vi "manual test UI.vi"(8 "error in (no error)":errorcluster caption="Fehler (Eingang, kein Fehler)", 11 "Spannungseinbruch Eingang":refnum<class "Spannungseinbruch.lvclass"> caption="DNL_LabVIEW Object in") -> (0 "error out":errorcluster caption="Fehler (Ausgang)", 1 "abbrechen":bool, 2 "Parameters":u32[](array[numeric]), 3 "Spannungseinbruch Ausgang":refnum<class "Spannungseinbruch.lvclass"> caption="DNL_LabVIEW Object out")   [LabVIEW 2013, in "Spannungseinbruch.lvclass"]
uses:
  Spannungseinbruch.lvclass
  Devices/CEG4500/ceg_make_cutofftest_states.ctl
panel:
  out "parameters":string[](array[string])
  in  "Parameters 2":u32[](array[numeric])
  in  "Testbeschreibung":string
  out "col":i32=3
  in  "abbrechen":bool
  in  "0 2":bool=TRUE
  in  "315 2":bool=TRUE
  in  "270 2":bool=TRUE
  in  "225 2":bool=TRUE
  in  "180 2":bool=TRUE
  in  "135 2":bool=TRUE
  in  "90 2":bool=TRUE
  in  "45 2":bool=TRUE
  in  "500ms 2":bool=TRUE
  in  "200ms 2":bool=TRUE
  in  "20ms 2":bool=TRUE
  in  "5000ms 2":bool=TRUE
  in  "erstellen":bool
  in  "COUNTER (1 - 999)":i32=5 min=0 max=999
  out "Str_counter":string
  in  "REP TIME (1-999s)":i32 min=1 max=999
  out "Str_reptime":string
  out "Commandlist":string
  out "parameter table":string[][](table)
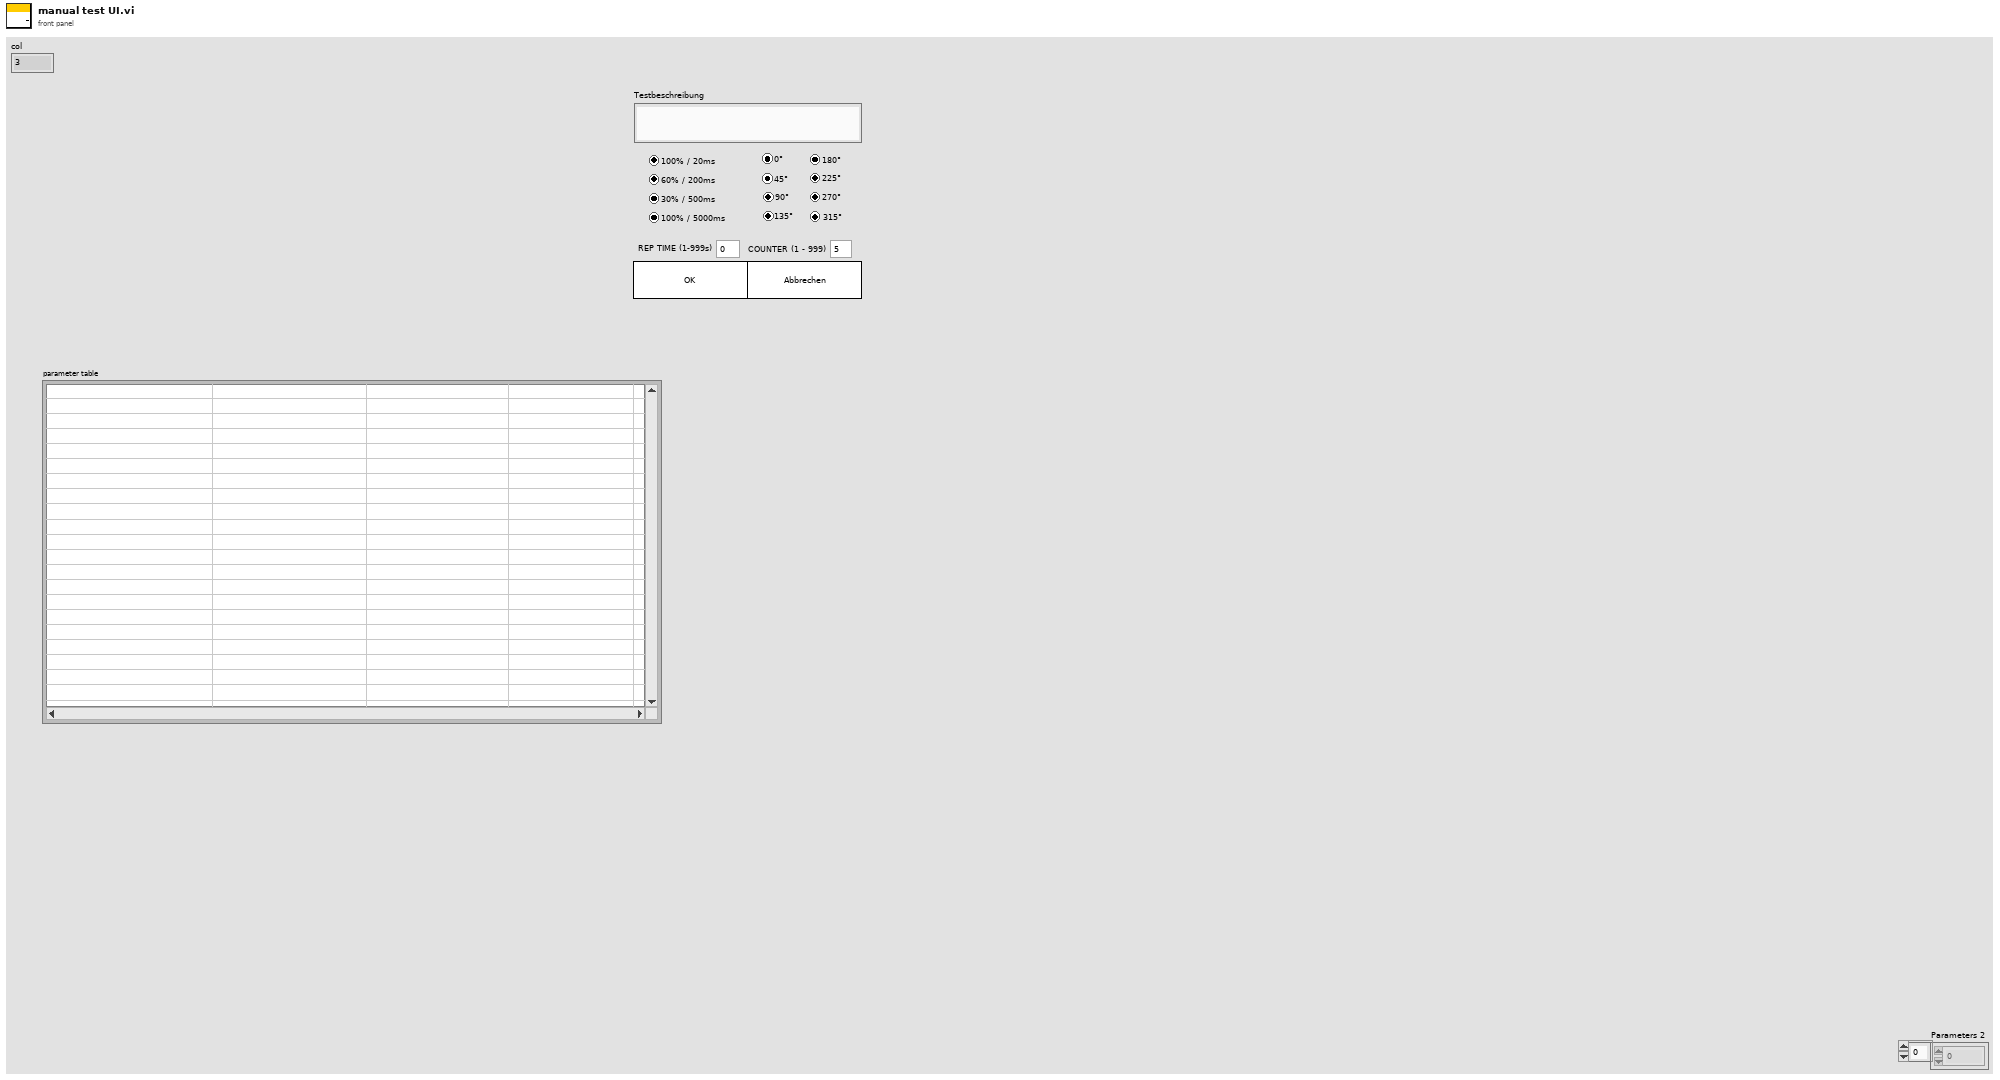
[diagram p1: front panel]
types:
  T1 = typedef "Spannungseinbruch.lvclass/ceg_make_cutofftest_states.ctl" = enum16{"make last test", "end", "make cmd strings", "make num strings", "start"}
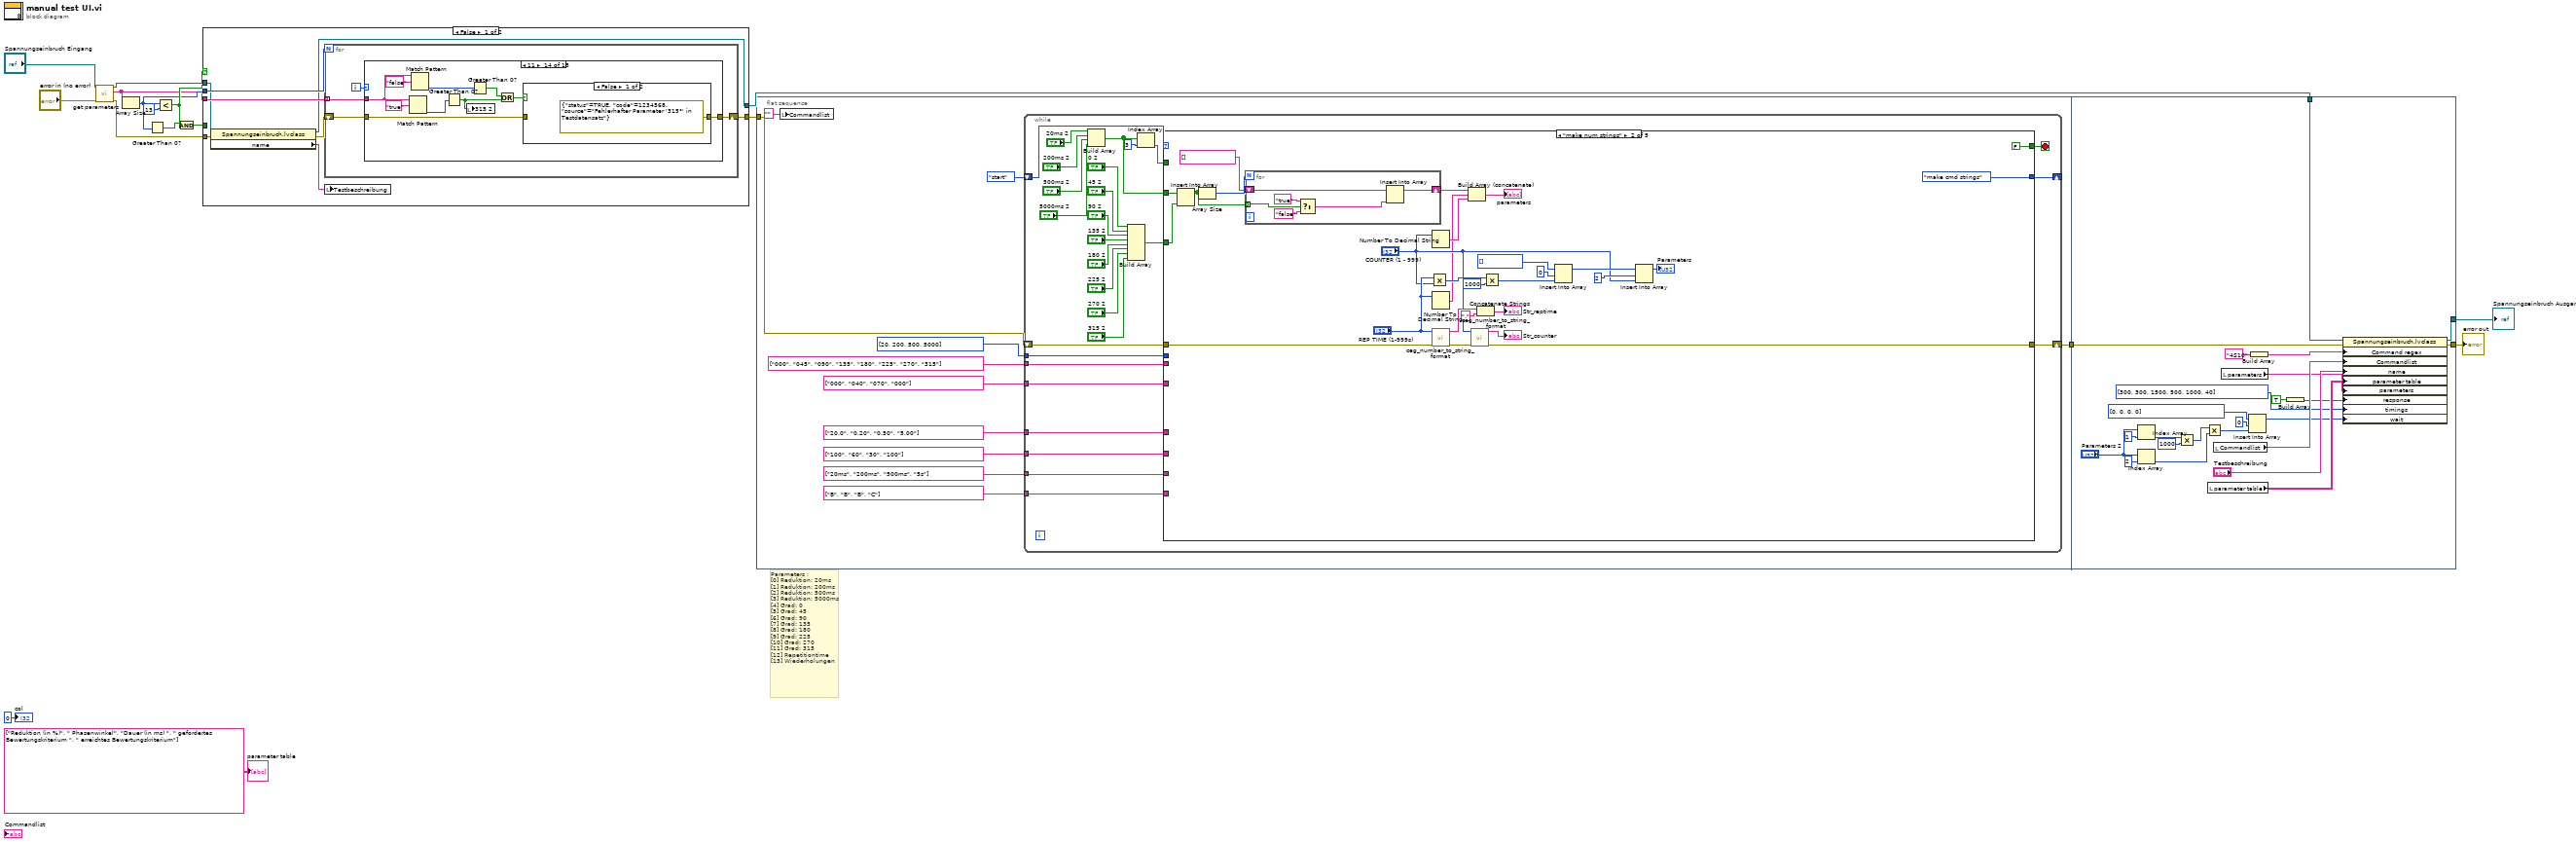
[diagram p0: block diagram]
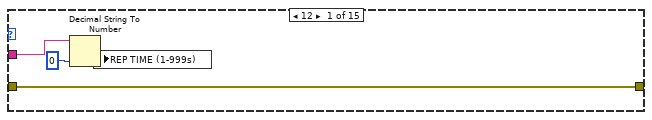
[diagram p2: hidden frame]
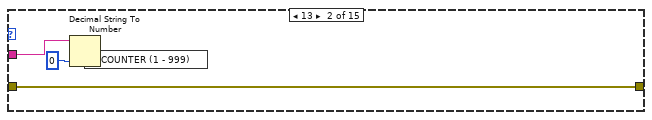
[diagram p3: hidden frame]
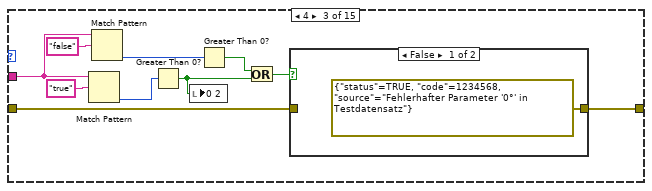
[diagram p4: hidden frame]
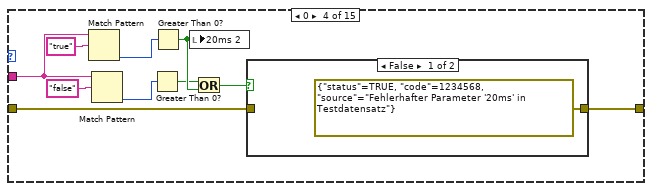
[diagram p6: hidden frame]
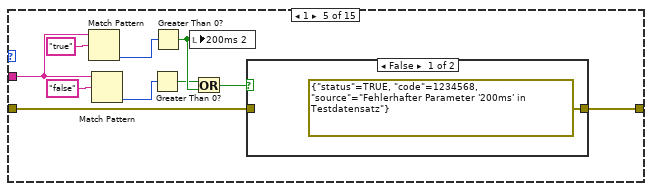
[diagram p8: hidden frame]
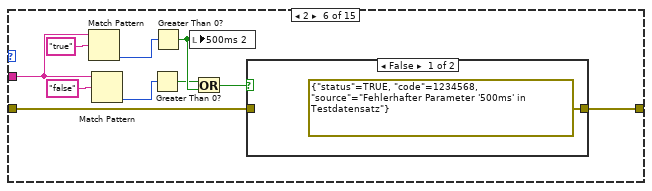
[diagram p10: hidden frame]
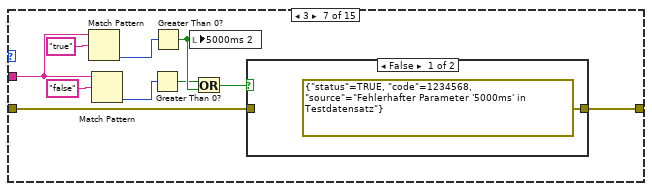
[diagram p12: hidden frame]
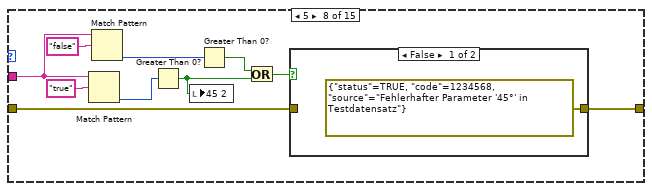
[diagram p14: hidden frame]
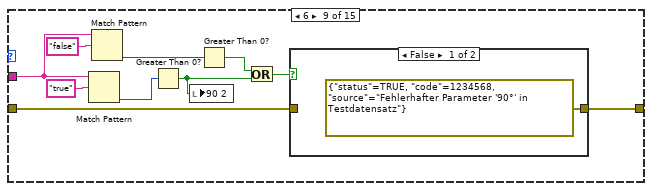
[diagram p16: hidden frame]
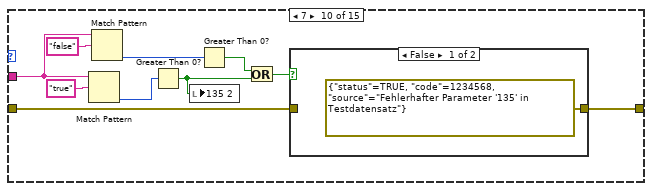
[diagram p18: hidden frame]
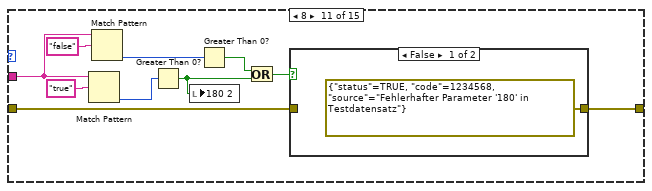
[diagram p20: hidden frame]
diagram:
  # "Parameters :\n[0] Reduktion: 20ms\n[1] Reduktion: 200ms\n[2] Reduktion: 500ms\n[3] Reduktion: 5000ms\n[4] Grad: 0\n[5] Grad: 45\n[6] Grad: 90\n[7] Grad: 135\n[8] Grad: 180\n[9] Grad: 225\n[10] Grad: 270\n[11] Grad: 315\n[12] Repetitiontime\n[13] Wiederholungen"
  n1 = call-dynamic "get parameters.vi"("error in (no error)"="error in (no error)", "TestInterface (Eingang)"="Spannungseinbruch Eingang") -> ("error out"=w7:errorcluster, "parameters"=w6:string[], "TestInterface (Ausgang)"=w13:refnum<class "Spannungseinbruch.lvclass">)  [unwired: 7 in]
  n2 = Array Size(array=w6) -> (size(s)=w9:i32)
  n3 = Greater Than 0?(x=w9) -> (x > 0?=w10:bool)
  n4 = Less?(x=w9, y=13) -> (x < y?=w11:bool)
  n5 = And(x=w10, y=w11) -> (x .and. y?=w12:bool)
  n6 = case shown="False" w11 {
    tunnel: w9 -> [w25 _]
    tunnel: w6 -> [w24 _]
    tunnel: w7 -> [w21 w186]
    tunnel: [w23 w184] -> w1
    tunnel: w12 -> [_ w185]
    tunnel: w13 -> [w22 w183]
    tunnel: [w18 w183] -> w3
    frame False {
      n7 = property class="Spannungseinbruch.lvclass"(reference=w22, error in=w21) -> (reference out=w18:refnum<class "Spannungseinbruch.lvclass">, error out=w20:errorcluster, "name"=w19:string)
      n8 = for {
        N: w25 -> [_]
        tunnel: w24 -> [w28] mode=indexing
        shift-right: [w27] -> w23
        shift-left: w20 -> [w26]
        i -> [w29]
        n9 = case shown="11" w29 {
          tunnel: w28 -> [w33 w37 w38 w50 w62 w74 w86 w98 w110 w122 w134 w146 w158 w170 _]
          tunnel: w26 -> [w30 w34 w40 w52 w64 w76 w88 w100 w112 w124 w136 w148 w160 w172 _]
          tunnel: [w30 w34 w42 w54 w66 w78 w90 w102 w114 w126 w138 w150 w162 w174 errorcluster {"status"=TRUE, "code"=1234567, "source"="zu viele Parameter für Test"} ("error constant")] -> w27
          frame 12 {
            n10 = Decimal String To Number(string=w33, default (0L)=u32 0 ("default (0 I32)")) -> (number=w32:u32)  [unwired: 1 in, 1 out]
            n11 = local write "REP TIME (1-999s)"(w32) -> ()
          }
          frame 13 {
            n12 = Decimal String To Number(string=w37, default (0L)=u32 0 ("default (0 I32)")) -> (number=w36:u32)  [unwired: 1 in, 1 out]
            n13 = local write "COUNTER (1 - 999)"(w36) -> ()
          }
          frame 4 {
            n14 = Match Pattern(string=w38, regular expression="true") -> (offset past match=w46:i32)  [unwired: 1 in, 3 out]
            n15 = Match Pattern(string=w38, regular expression="false") -> (offset past match=w44:i32)  [unwired: 1 in, 3 out]
            n16 = Greater Than 0?(x=w46) -> (x > 0?=w43:bool)
            n17 = local write "0 2"(w43) -> ()
            n18 = Greater Than 0?(x=w44) -> (x > 0?=w41:bool)
            n19 = Or(x=w41, y=w43) -> (x .or. y?=w39:bool)
            n20 = case shown="False" w39 {
              tunnel: [errorcluster {"status"=TRUE, "code"=1234568, "source"="Fehlerhafter Parameter '0°' in Testdatensatz"} ("error constant") w49] -> w42
              tunnel: w40 -> [_ w49]
              frame False {
              }
              frame True {
              }
            }
          }
          frame 0 {
            n21 = Match Pattern(string=w50, regular expression="true") -> (offset past match=w58:i32)  [unwired: 1 in, 3 out]
            n22 = Match Pattern(string=w50, regular expression="false") -> (offset past match=w56:i32)  [unwired: 1 in, 3 out]
            n23 = Greater Than 0?(x=w56) -> (x > 0?=w53:bool)
            n24 = Greater Than 0?(x=w58) -> (x > 0?=w55:bool)
            n25 = local write "20ms 2"(w55) -> ()
            n26 = Or(x=w53, y=w55) -> (x .or. y?=w51:bool)
            n27 = case shown="False" w51 {
              tunnel: [errorcluster {"status"=TRUE, "code"=1234568, "source"="Fehlerhafter Parameter '20ms' in Testdatensatz"} ("error constant") w61] -> w54
              tunnel: w52 -> [_ w61]
              frame False {
              }
              frame True {
              }
            }
          }
          frame 1 {
            n28 = Match Pattern(string=w62, regular expression="true") -> (offset past match=w70:i32)  [unwired: 1 in, 3 out]
            n29 = Match Pattern(string=w62, regular expression="false") -> (offset past match=w68:i32)  [unwired: 1 in, 3 out]
            n30 = Greater Than 0?(x=w68) -> (x > 0?=w65:bool)
            n31 = Greater Than 0?(x=w70) -> (x > 0?=w67:bool)
            n32 = local write "200ms 2"(w67) -> ()
            n33 = Or(x=w65, y=w67) -> (x .or. y?=w63:bool)
            n34 = case shown="False" w63 {
              tunnel: [errorcluster {"status"=TRUE, "code"=1234568, "source"="Fehlerhafter Parameter '200ms' in Testdatensatz"} ("error constant") w73] -> w66
              tunnel: w64 -> [_ w73]
              frame False {
              }
              frame True {
              }
            }
          }
          frame 2 {
            n35 = Match Pattern(string=w74, regular expression="true") -> (offset past match=w82:i32)  [unwired: 1 in, 3 out]
            n36 = Match Pattern(string=w74, regular expression="false") -> (offset past match=w80:i32)  [unwired: 1 in, 3 out]
            n37 = Greater Than 0?(x=w80) -> (x > 0?=w77:bool)
            n38 = Greater Than 0?(x=w82) -> (x > 0?=w79:bool)
            n39 = local write "500ms 2"(w79) -> ()
            n40 = Or(x=w77, y=w79) -> (x .or. y?=w75:bool)
            n41 = case shown="False" w75 {
              tunnel: [errorcluster {"status"=TRUE, "code"=1234568, "source"="Fehlerhafter Parameter '500ms' in Testdatensatz"} ("error constant") w85] -> w78
              tunnel: w76 -> [_ w85]
              frame False {
              }
              frame True {
              }
            }
          }
          frame 3 {
            n42 = Match Pattern(string=w86, regular expression="true") -> (offset past match=w94:i32)  [unwired: 1 in, 3 out]
            n43 = Match Pattern(string=w86, regular expression="false") -> (offset past match=w92:i32)  [unwired: 1 in, 3 out]
            n44 = Greater Than 0?(x=w92) -> (x > 0?=w89:bool)
            n45 = Greater Than 0?(x=w94) -> (x > 0?=w91:bool)
            n46 = local write "5000ms 2"(w91) -> ()
            n47 = Or(x=w89, y=w91) -> (x .or. y?=w87:bool)
            n48 = case shown="False" w87 {
              tunnel: [errorcluster {"status"=TRUE, "code"=1234568, "source"="Fehlerhafter Parameter '5000ms' in Testdatensatz"} ("error constant") w97] -> w90
              tunnel: w88 -> [_ w97]
              frame False {
              }
              frame True {
              }
            }
          }
          frame 5 {
            n49 = Match Pattern(string=w98, regular expression="true") -> (offset past match=w106:i32)  [unwired: 1 in, 3 out]
            n50 = Match Pattern(string=w98, regular expression="false") -> (offset past match=w104:i32)  [unwired: 1 in, 3 out]
            n51 = Greater Than 0?(x=w106) -> (x > 0?=w103:bool)
            n52 = local write "45 2"(w103) -> ()
            n53 = Greater Than 0?(x=w104) -> (x > 0?=w101:bool)
            n54 = Or(x=w101, y=w103) -> (x .or. y?=w99:bool)
            n55 = case shown="False" w99 {
              tunnel: [errorcluster {"status"=TRUE, "code"=1234568, "source"="Fehlerhafter Parameter '45°' in Testdatensatz"} ("error constant") w109] -> w102
              tunnel: w100 -> [_ w109]
              frame False {
              }
              frame True {
              }
            }
          }
          frame 6 {
            n56 = Match Pattern(string=w110, regular expression="true") -> (offset past match=w118:i32)  [unwired: 1 in, 3 out]
            n57 = Match Pattern(string=w110, regular expression="false") -> (offset past match=w116:i32)  [unwired: 1 in, 3 out]
            n58 = Greater Than 0?(x=w118) -> (x > 0?=w115:bool)
            n59 = local write "90 2"(w115) -> ()
            n60 = Greater Than 0?(x=w116) -> (x > 0?=w113:bool)
            n61 = Or(x=w113, y=w115) -> (x .or. y?=w111:bool)
            n62 = case shown="False" w111 {
              tunnel: [errorcluster {"status"=TRUE, "code"=1234568, "source"="Fehlerhafter Parameter '90°' in Testdatensatz"} ("error constant") w121] -> w114
              tunnel: w112 -> [_ w121]
              frame False {
              }
              frame True {
              }
            }
          }
          frame 7 {
            n63 = Match Pattern(string=w122, regular expression="true") -> (offset past match=w130:i32)  [unwired: 1 in, 3 out]
            n64 = Match Pattern(string=w122, regular expression="false") -> (offset past match=w128:i32)  [unwired: 1 in, 3 out]
            n65 = Greater Than 0?(x=w130) -> (x > 0?=w127:bool)
            n66 = local write "135 2"(w127) -> ()
            n67 = Greater Than 0?(x=w128) -> (x > 0?=w125:bool)
            n68 = Or(x=w125, y=w127) -> (x .or. y?=w123:bool)
            n69 = case shown="False" w123 {
              tunnel: [errorcluster {"status"=TRUE, "code"=1234568, "source"="Fehlerhafter Parameter '135' in Testdatensatz"} ("error constant") w133] -> w126
              tunnel: w124 -> [_ w133]
              frame False {
              }
              frame True {
              }
            }
          }
          frame 8 {
            n70 = Match Pattern(string=w134, regular expression="true") -> (offset past match=w142:i32)  [unwired: 1 in, 3 out]
            n71 = Match Pattern(string=w134, regular expression="false") -> (offset past match=w140:i32)  [unwired: 1 in, 3 out]
            n72 = Greater Than 0?(x=w142) -> (x > 0?=w139:bool)
            n73 = local write "180 2"(w139) -> ()
            n74 = Greater Than 0?(x=w140) -> (x > 0?=w137:bool)
            n75 = Or(x=w137, y=w139) -> (x .or. y?=w135:bool)
            n76 = case shown="False" w135 {
              tunnel: [errorcluster {"status"=TRUE, "code"=1234568, "source"="Fehlerhafter Parameter '180' in Testdatensatz"} ("error constant") w145] -> w138
              tunnel: w136 -> [_ w145]
              frame False {
              }
              frame True {
              }
            }
          }
          frame 9 {
            n77 = Match Pattern(string=w146, regular expression="true") -> (offset past match=w154:i32)  [unwired: 1 in, 3 out]
            n78 = Match Pattern(string=w146, regular expression="false") -> (offset past match=w152:i32)  [unwired: 1 in, 3 out]
            n79 = Greater Than 0?(x=w154) -> (x > 0?=w151:bool)
            n80 = local write "225 2"(w151) -> ()
            n81 = Greater Than 0?(x=w152) -> (x > 0?=w149:bool)
            n82 = Or(x=w149, y=w151) -> (x .or. y?=w147:bool)
            n83 = case shown="False" w147 {
              tunnel: [errorcluster {"status"=TRUE, "code"=1234568, "source"="Fehlerhafter Parameter '225°' in Testdatensatz"} ("error constant") w157] -> w150
              tunnel: w148 -> [_ w157]
              frame False {
              }
              frame True {
              }
            }
          }
          frame 10 {
            n84 = Match Pattern(string=w158, regular expression="true") -> (offset past match=w166:i32)  [unwired: 1 in, 3 out]
            n85 = Match Pattern(string=w158, regular expression="false") -> (offset past match=w164:i32)  [unwired: 1 in, 3 out]
            n86 = Greater Than 0?(x=w166) -> (x > 0?=w163:bool)
            n87 = local write "270 2"(w163) -> ()
            n88 = Greater Than 0?(x=w164) -> (x > 0?=w161:bool)
            n89 = Or(x=w161, y=w163) -> (x .or. y?=w159:bool)
            n90 = case shown="False" w159 {
              tunnel: [errorcluster {"status"=TRUE, "code"=1234568, "source"="Fehlerhafter Parameter '270°' in Testdatensatz"} ("error constant") w169] -> w162
              tunnel: w160 -> [_ w169]
              frame False {
              }
              frame True {
              }
            }
          }
          frame 11 {
            n91 = Match Pattern(string=w170, regular expression="true") -> (offset past match=w178:i32)  [unwired: 1 in, 3 out]
            n92 = Match Pattern(string=w170, regular expression="false") -> (offset past match=w176:i32)  [unwired: 1 in, 3 out]
            n93 = Greater Than 0?(x=w178) -> (x > 0?=w175:bool)
            n94 = local write "315 2"(w175) -> ()
            n95 = Greater Than 0?(x=w176) -> (x > 0?=w173:bool)
            n96 = Or(x=w173, y=w175) -> (x .or. y?=w171:bool)
            n97 = case shown="False" w171 {
              tunnel: [errorcluster {"status"=TRUE, "code"=1234568, "source"="Fehlerhafter Parameter '315°' in Testdatensatz"} ("error constant") w181] -> w174
              tunnel: w172 -> [_ w181]
              frame False {
              }
              frame True {
              }
            }
          }
          frame 14, Default {
          }
        }
      }
      n98 = local write "Testbeschreibung"(w19) -> ()
    }
    frame True {
      n99 = case shown="False" w185 {
        tunnel: w186 -> [w192 _]
        tunnel: [w192 errorcluster {"status"=TRUE, "code"=123458, "source"="Der Parametersatz für den aktuellen Test ist unvollständig und\nkonnte nicht geladen werden"} ("error constant")] -> w184
        frame False {
        }
        frame True {
        }
      }
      n100 = Get Date/Time In Seconds() -> (seconds since 1Jan1904=w191:timestamp)
      n101 = Format Date/Time String(time format string (%c)="%d.%m %H:%M" ("Zeitformatierungs-String (%c)"), seconds (now)=w191) -> (date/time string=w188:string)  [unwired: 1 in]
      n102 = Concatenate Strings("Benutzerdefinierter Test vom " ("name"), w188) -> (w187:string)
      n103 = local write "Testbeschreibung"(w187) -> ()
    }
  }
  n104 = flat-sequence {
    tunnel: w1 -> [w199]
    tunnel: [w200] -> w15
    tunnel: [w389] -> w17
    tunnel: w15 -> [w410]
    tunnel: w3 -> [w412]
    tunnel: [w409] -> w5
    frame #0 {
      n105 = local write "Commandlist"("" ("Commandlist")) -> ()
      n106 = while {
        tunnel: string[] ["000", "040", "070", "000"] -> [w230]
        tunnel: string[] ["000", "045", "090", "135", "180", "225", "270", "315"] -> [w229]
        tunnel: string[] ["20.0", "0.20", "0.50", "5.00"] -> [w228]
        shift-right: [w227] -> w200
        shift-left: w199 -> [w232]
        shift-right: [w226] -> _
        shift-left: ceg_make_cutofftest_states."start" -> [w231]
        tunnel: string[] ["20ms", "200ms", "500ms", "5s"] -> [w224]
        tunnel: string[] ["100", "60", "30", "100"] -> [w207]
        tunnel: string[] ["B", "B", "B", "C"] -> [w206]
        tunnel: u32[] [20, 200, 500, 5000] -> [w205]
        stop <- w225 stop-if-true
        n107 = Build Array("20ms 2", "200ms 2", "500ms 2", "5000ms 2") -> (w208:bool[])
        n108 = Build Array("0 2", "45 2", "90 2", "135 2", "180 2", "225 2", "270 2", "315 2") -> (w215:bool[])
        n109 = Index Array(array=w208, index=3) -> (element=w209:bool)
        n110 = case shown="\"make num strings\"" w231 {
          tunnel: w232 -> [w236 w290 w302 w314 w388]
          tunnel: w230 -> [_ _ _ w320 _]
          tunnel: w229 -> [_ _ _ w319 _]
          tunnel: w228 -> [_ _ _ w318 _]
          tunnel: w208 -> [_ w273 _ w309 _]
          tunnel: w209 -> [w234 _ _ w317 _]
          tunnel: [w236 w289 w302 w314 w388] -> w227
          tunnel: [ceg_make_cutofftest_states."end" ceg_make_cutofftest_states."make cmd strings" w304 ceg_make_cutofftest_states."make last test" ceg_make_cutofftest_states."end"] -> w226
          tunnel: [FALSE FALSE FALSE FALSE TRUE] -> w225
          tunnel: w215 -> [_ w272 _ w308 _]
          tunnel: w224 -> [_ _ _ w313 _]
          tunnel: w207 -> [_ _ _ w312 _]
          tunnel: w206 -> [_ _ _ w311 _]
          tunnel: w205 -> [_ _ _ w310 _]
          frame "make last test", Default {
            n111 = case shown="True" w234 {
              frame False {
              }
              frame True {
                w242 = "\r\n"
                n112 = local read "parameter table"() -> (w255:string[][])
                n113 = local read "Commandlist"() -> (w267:string)
                n114 = local read "Str_counter"() -> (w264:string)
                n115 = local read "Str_reptime"() -> (w262:string)
                n116 = local read "Parameters"() -> (w239:u32[])
                n117 = local read "col"() -> (w251:i32)
                n118 = Increment(x=w251) -> (x+1=w244:i32)
                n119 = Insert Into Array(array=w239, index=1, new element=u32 5000 ("new element/subarray")) -> (w240:u32[])
                n120 = Concatenate Strings(w267, "3A" ("string"), "000" ("string"), w264, "000" ("string"), w262, "5.00" ("string"), "000." ("string"), w242, "3S10" ("string"), w242, "3y" ("string"), w242) -> (w266:string)
                n121 = Replace Array Subset(array=w255, new element="0" ("new element/subarray"), index (row)=1, index (col)=w244) -> (w250:string[][])
                n122 = local write "Commandlist"(w266) -> ()
                n123 = local write "Parameters"(w240) -> ()
                n124 = Replace Array Subset(array=w250, new element="5s" ("new element/subarray"), index (row)=2, index (col)=w244) -> (w249:string[][])
                n125 = Replace Array Subset(array=w249, new element="100" ("new element/subarray"), index (row)=0, index (col)=w244) -> (w245:string[][])
                n126 = Replace Array Subset(array=w245, new element="C" ("new element/subarray"), index (row)=3, index (col)=w244) -> (w246:string[][])
                n127 = local write "parameter table"(w246) -> ()
              }
            }
          }
          frame "make num strings" {
            n128 = Insert Into Array(array=w273, new element=w272) -> (w275:bool[])  [unwired: 1 in]
            n129 = Array Size(array=w275) -> (size(s)=w276:i32)
            n130 = for {
              N: w276 -> [_]
              tunnel: w275 -> [w301] mode=indexing
              shift-right: [w296] -> w271
              shift-left: string[] [] -> [w297]
              n131 = Select(t="true", s=w301, f="false") -> (s? t:f=w298:string)
              n132 = Insert Into Array(array=w297, new element=w298) -> (w296:string[])  [unwired: 1 in]
            }
            n133 = Multiply(x="REP TIME (1-999s)", y="COUNTER (1 - 999)") -> (x*y=w286:i32)
            n134 = Number To Decimal String(number="COUNTER (1 - 999)") -> (decimal integer string=w269:string)  [unwired: 1 in]
            n135 = Number To Decimal String(number="REP TIME (1-999s)") -> (decimal integer string=w268:string)  [unwired: 1 in]
            n136 = call "ceg_number_to_string_format.vi"("Counter"="REP TIME (1-999s)", "erro in"=w290) -> ("out"=w293:string, "error out"=w292:errorcluster)  [unwired: 7 in]
            n137 = Build Array (concatenate)(w271, w268, w269) -> (→"parameters":string[])
            n138 = call "ceg_number_to_string_format.vi"("Counter"="COUNTER (1 - 999)", "erro in"=w292) -> ("out"=→"Str_counter":string, "error out"=w289:errorcluster)  [unwired: 7 in]
            n139 = Concatenate Strings(w293, "." ("string")) -> (→"Str_reptime":string)
            n140 = Multiply(x=w286, y=1000) -> (x*y=w284:i32)
            n141 = Insert Into Array(array=u32[] [] ("Parameters"), index=0, new element=w284) -> (w280:u32[])
            n142 = Insert Into Array(array=w280, index=2, new element="COUNTER (1 - 999)") -> (→"Parameters":u32[])
          }
          frame "start" {
            n143 = event shown="[1] \"abbrechen\": Value Change" {
              selector: _ -> [_ _]
              dyn-events: _ -> [_ _]
              timeout: _ -> [_ _]
              tunnel: [ceg_make_cutofftest_states."make num strings" ceg_make_cutofftest_states."end"] -> w304
              event "erstellen": Value Change {
                n144 = event-data() -> ()  [unwired: 1 in, 6 out]
              }
              event "abbrechen": Value Change {
                n145 = event-data() -> ()  [unwired: 1 in, 6 out]
                "abbrechen" <- "abbrechen"
              }
            }
          }
          frame "make cmd strings" {
            n146 = for {
              N: 3 -> [_]
              tunnel: w317 -> [_]
              tunnel: w309 -> [w328] mode=indexing
              tunnel: w320 -> [w331] mode=indexing
              tunnel: w319 -> [w330]
              tunnel: w318 -> [w329] mode=indexing
              tunnel: w308 -> [w327]
              tunnel: w313 -> [w325] mode=indexing
              tunnel: w312 -> [w324] mode=indexing
              tunnel: w311 -> [w323] mode=indexing
              tunnel: w310 -> [w322] mode=indexing
              i -> [w326]
              n147 = case shown="True" w328 {
                tunnel: w327 -> [_ w353]
                tunnel: w331 -> [_ w352]
                tunnel: w330 -> [_ w351]
                tunnel: w329 -> [_ w350]
                tunnel: w326 -> [_ _]
                tunnel: w325 -> [_ w345]
                tunnel: w324 -> [_ w349]
                tunnel: w323 -> [_ w341]
                tunnel: w322 -> [_ w338]
                frame False {
                }
                frame True {
                  n148 = local read "col"() -> (w346:i32)
                  n149 = local read "parameter table"() -> (w335:string[][])
                  n150 = Increment(x=w346) -> (x+1=w333:i32)
                  n151 = local read "Parameters"() -> (w339:u32[])
                  n152 = local write "col"(w333) -> ()
                  n153 = for {
                    N: 8 -> [_]
                    tunnel: w353 -> [w359] mode=indexing
                    tunnel: w352 -> [w358]
                    tunnel: w351 -> [w357] mode=indexing
                    tunnel: w350 -> [w356]
                    tunnel: w333 -> [w355]
                    n154 = case shown="True" w359 {
                      tunnel: w358 -> [_ w380]
                      tunnel: w357 -> [_ w367]
                      tunnel: w356 -> [_ w374]
                      tunnel: w355 -> [_ w365]
                      frame False {
                      }
                      frame True {
                        w364 = 1 ("disabled index (col)")
                        w361 = "\r\n"
                        n155 = local read "parameter table"() -> (w368:string[][])
                        n156 = local read "Commandlist"() -> (w379:string)
                        n157 = local read "Str_counter"() -> (w376:string)
                        n158 = local read "Str_reptime"() -> (w373:string)
                        n159 = Index Array(array=w368, index (row)=w364, index (col)=w365) -> (element=w369:string)
                        n160 = Concatenate Strings(w379, "3A" ("string"), w380, w376, w367, w373, w374, "000." ("string"), w361, "3a" ("string"), w361, "3S10" ("string"), w361, "3y" ("string"), w361) -> (w378:string)
                        n161 = String Length(string=w369) -> (length=w370:i32)
                        n162 = Greater Than 0?(x=w370) -> (x > 0?=w371:bool)
                        n163 = local write "Commandlist"(w378) -> ()
                        n164 = case shown="True" w371 {
                          tunnel: w369 -> [_ w385]
                          tunnel: w367 -> [w381 w383]
                          tunnel: [w381 w382] -> w366
                          frame False {
                          }
                          frame True {
                            n165 = Concatenate Strings(w385, "," ("string"), w383) -> (w382:string)
                          }
                        }
                        n166 = Replace Array Subset(array=w368, new element=w366, index (row)=w364, index (col)=w365) -> (w372:string[][])
                        n167 = local write "parameter table"(w372) -> ()
                      }
                    }
                  }
                  n168 = Insert Into Array(array=w335, index (col)=w333, new element=string[][] [[""], [""], [""], [""], [""]]) -> (w332:string[][])  [unwired: 1 in]
                  n169 = Replace Array Subset(array=w339, new element=w338, index=1) -> (w336:u32[])
                  n170 = local write "Parameters"(w336) -> ()
                  n171 = Replace Array Subset(array=w332, new element=w349, index (row)=0 ("disabled index (col)"), index (col)=w333) -> (w344:string[][])
                  n172 = Replace Array Subset(array=w344, new element=w345, index (row)=2 ("disabled index (col)"), index (col)=w333) -> (w342:string[][])
                  n173 = Replace Array Subset(array=w342, new element=w341, index (row)=3 ("disabled index (col)"), index (col)=w333) -> (w340:string[][])
                  n174 = local write "parameter table"(w340) -> ()
                }
              }
            }
          }
          frame "end" {
          }
        }
      }
    }
    frame #1 {
      n175 = Index Array(array="Parameters 2", index=1) -> (element=w398:u32)
      n176 = Index Array(array="Parameters 2", index=2) -> (element=w404:u32)
      n177 = Multiply(x=w398, y=u32 1000) -> (x*y=w405:u32)
      n178 = Multiply(x=w405, y=w404) -> (x*y=w406:u32)
      n179 = local read "parameter table"() -> (w408:string[][])
      n180 = local read "Commandlist"() -> (w407:string)
      n181 = local read "parameters"() -> (w390:string[])
      n182 = Insert Into Array(array=i32[] [0, 0, 0, 0] ("Timings"), index=0, new element=w406) -> (w395:i32[])
      n183 = Build Array("4S10") -> (w391:string[])
      n184 = Build Array(TRUE) -> (w392:bool[])
      n185 = property class="Spannungseinbruch.lvclass"(reference=w412, error in=w410, "Command regex"=w391, "Commandlist"=w407, "name"="Testbeschreibung", "parameter table"=w408, "parameters"=w390, "response"=w392, "timings"=u32[] [300, 300, 1500, 500, 1000, 40] ("Timings"), "wait"=w395) -> (reference out=w409:refnum<class "Spannungseinbruch.lvclass">, error out=w389:errorcluster)
    }
  }
  "error out" <- w17
  "parameter table" <- string[][] [["Reduktion (in %)"], [" Phasenwinkel"], ["Dauer (in ms) "], [" gefordertes Bewertungskriterium "], [" erreichtes Bewertungskriterium"]]
  "col" <- 0 ("numberofTests")
  "Spannungseinbruch Ausgang" <- w5
